vi "Write Init Mouse.vi"(8 "error in (no error)":errorcluster, 10 "Init Mouse":timestamp, 11 "Mouse in":refnum<class "Mouse.lvclass">) -> (0 "error out":errorcluster, 3 "Mouse out":refnum<class "Mouse.lvclass">)   [LabVIEW 2021, in "Mouse.lvclass"]
uses:
  Mouse.lvclass
  Mouse.lvclass/Mouse.ctl
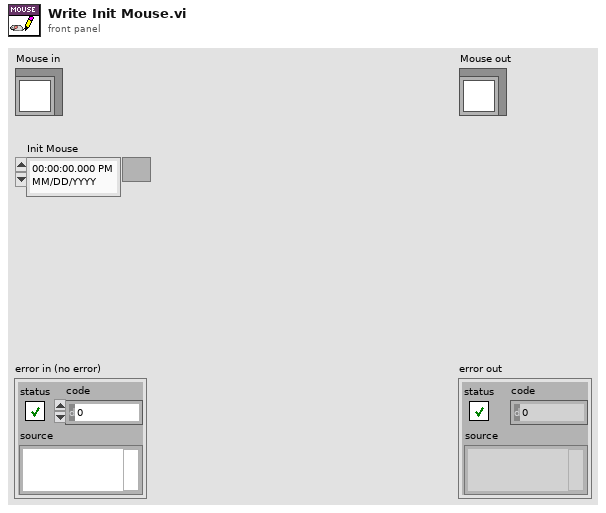
[diagram p1: front panel]
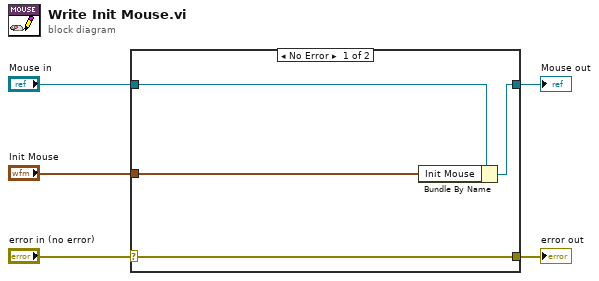
[diagram p0: block diagram]
diagram:
  n1 = case shown="No Error" "error in (no error)" {
    selector: "error in (no error)" -> [w9 w10]
    tunnel: [w9 w10] -> w4
    tunnel: [w7 w11] -> w2
    tunnel: "Mouse in" -> [w8 w11]
    tunnel: "Init Mouse" -> [w6 _]
    frame No Error {
      n2 = Bundle By Name(cluster=w8, "Init Mouse"=w6) -> (w7:refnum<class "Mouse.lvclass">)
    }
    frame Error {
    }
  }
  "error out" <- w4
  "Mouse out" <- w2
